vi "test BM Disable.vi"(8 "error in (no error)":errorcluster, 11 "BM Enable in":refnum<class "BM Enable.lvclass">) -> (0 "error out":errorcluster, 3 "BM Enable out":refnum<class "BM Enable.lvclass">)   [LabVIEW 2016, in "BM Enable.lvclass"]
uses:
  BM Enable.lvclass
  1553 Board/1553 Board.lvclass
  PPLs/FPGA Interface.lvlibp/FPGA Interface/FPGA Interface.lvclass
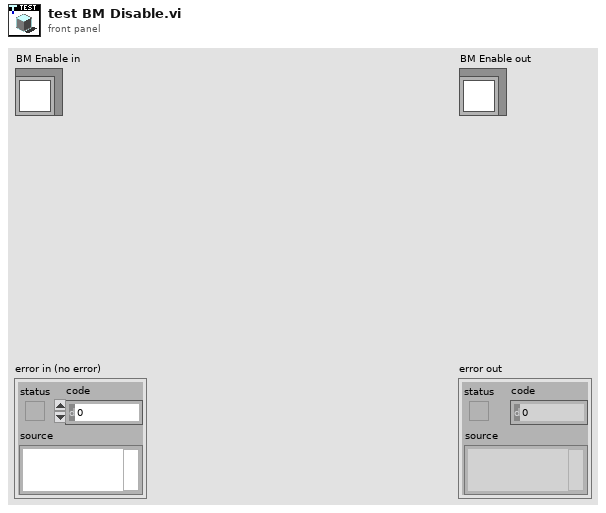
[diagram p1: front panel]
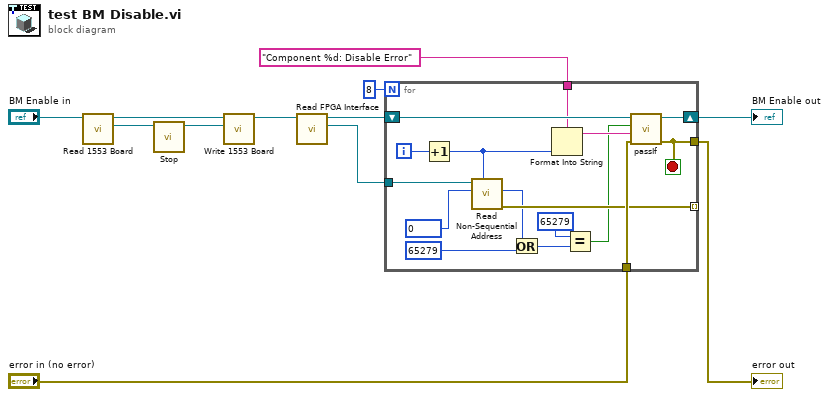
[diagram p0: block diagram]
diagram:
  n1 = call-dynamic "Read 1553 Board.vi"("1553 Test in"="BM Enable in") -> ("1553 Board"=w4:refnum<class "1553 Board.lvclass">, "1553 Test out"=w5:refnum<class "BM Enable.lvclass">)  [unwired: 8 in, 1 out]
  n2 = call-dynamic "Stop.vi"("1553 Board in"=w4) -> ("1553 Board out"=w3:refnum<class "1553 Board.lvclass">)  [unwired: 9 in, 1 out]
  n3 = call-dynamic "Write 1553 Board.vi"("1553 Board"=w3, "1553 Test in"=w5) -> ("1553 Test out"=w1:refnum<class "BM Enable.lvclass">)  [unwired: 8 in, 1 out]
  n4 = call-dynamic "Read FPGA Interface.vi"("1553 Test in"=w1) -> ("FPGA Interface"=w9:refnum<class "FPGA Interface.lvclass">, "1553 Test out"=w10:refnum<class "BM Enable.lvclass">)  [unwired: 8 in, 1 out]
  n5 = for {
    N: 8 -> [_]
    tunnel: w9 -> [w28]
    shift-right: [w24] -> w8
    shift-left: w10 -> [w25]
    tunnel: "Component %d: Disable Error" ("custom report message (\"\")") -> [w23]
    tunnel: "error in (no error)" -> [w20]
    tunnel: [w19] -> w6
    tunnel: [w18] -> _ mode=indexing
    i -> [w27]
    stop <- w19 stop-if-true
    n6 = Increment(x=w27) -> (x+1=w22:i32)
    n7 = call-dynamic "Read Non-Sequential Address.vi"("Target IC (1-8)"=w22, "Address"=u16 0, "FPGA Interface in"=w28) -> ("error out"=w18:errorcluster, "Data"=w15:u16)  [unwired: 7 in]
    n8 = Or(x=w15, y=u16 65279) -> (x .or. y?=w16:u16)
    n9 = Format Into String(format string=w23, w22) -> (resulting string=w21:string)  [unwired: 2 in, 1 out]
    n10 = Equal?(x=u16 65279, y=w16) -> (x = y?=w13:bool)
    n11 = call-dynamic "passIf.vi"("error in (no error)"=w20, "message (\"\")"=w21, "pass"=w13, "TestCase in"=w25) -> ("error out"=w19:errorcluster, "TestCase out"=w24:refnum<class "BM Enable.lvclass">)  [unwired: 6 in]
  }
  "error out" <- w6
  "BM Enable out" <- w8
